vi "multiplexer timing.vi"(2 "clock time in ms (25)":u32=25, 3 "Reset":bool=TRUE) -> (1 "Clock Tick":bool, 4 "Latch":bool, 6 "Total Running Time":u32, 7 "Time Since Tick":u32, 8 "Clock Counter":u32)   [LabVIEW 2014]
panel:
  in  "latch time in ms (10)":u32
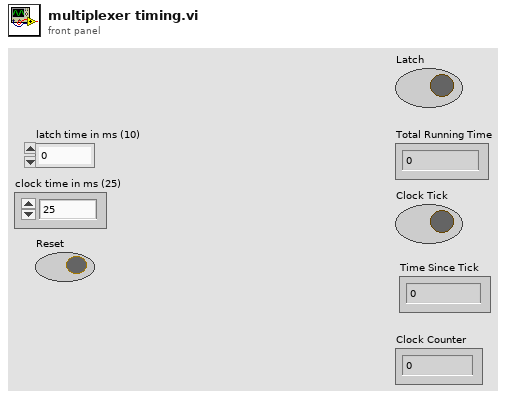
[diagram p1: front panel]
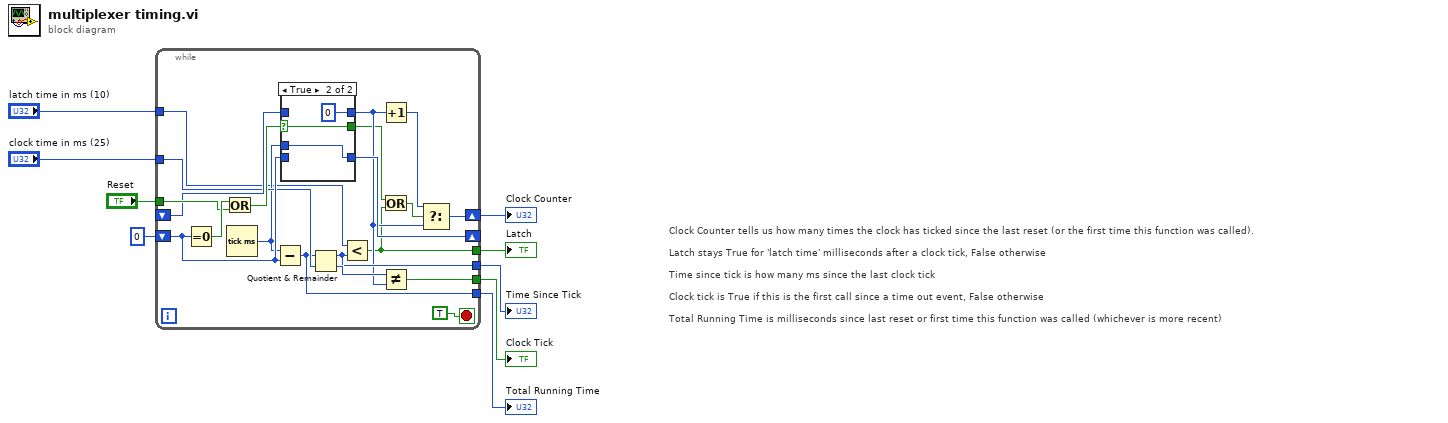
[diagram p0: block diagram]
diagram:
  # "Clock Counter tells us how many times the clock has ticked since the last reset (or the first time this function was called).\n\nLatch stays True for 'latch time' milliseconds after a clock tick, False otherwise\n\nTime since tick is how many ms since the last clock tick\n\nClock tick is True if this is the first call since a time out event, False otherwise\n\nTotal Running Time is milliseconds since last reset or first time this function was called (whichever is more recent)"
  n1 = while {
    shift-right: [w14] -> w3
    shift-left: _ -> [w22]
    shift-right: [w27] -> _
    shift-left: u32 0 -> [w26]
    tunnel: "Reset" -> [w24]
    tunnel: "clock time in ms (25)" -> [w21]
    tunnel: [w11] -> w6
    tunnel: [w18] -> w5
    tunnel: [w20] -> w4
    tunnel: "latch time in ms (10)" -> [w17]
    tunnel: [w13] -> w1
    stop <- TRUE stop-if-true
    n2 = Equal To 0?(x=w26) -> (x = 0?=w25:bool)
    n3 = Or(x=w25, y=w24) -> (x .or. y?=w23:bool)
    n4 = Tick Count (ms)() -> (millisecond timer value=w19:u32)
    n5 = Subtract(x=w19, y=w26) -> (x-y=w20:u32)
    n6 = case shown="True" w23 {
      selector: w23 -> [w30 w33]
      tunnel: [w32 w34] -> w27
      tunnel: w26 -> [w32 _]
      tunnel: w22 -> [w31 _]
      tunnel: [w31 u32 0 ("Clock Counter")] -> w15
      tunnel: w19 -> [_ w34]
      tunnel: [w30 w33] -> w12
      frame False {
      }
      frame True {
      }
    }
    n7 = Quotient & Remainder(x=w20, y=w21) -> (x-y*floor(x/y)=w18:u32, floor(x/y)=w29:u32)
    n8 = Less?(x=w17, y=w18) -> (x < y?=w13:bool)
    n9 = Increment(x=w15) -> (x+1=w16:u32)
    n10 = Or(x=w12, y=w13) -> (x .or. y?=w10:bool)
    n11 = Not Equal?(x=w29, y=w15) -> (x != y?=w11:bool)
    n12 = Select(t=w16, s=w10, f=w15) -> (s? t:f=w14:u32)
  }
  "Clock Counter" <- w3
  "Time Since Tick" <- w5
  "Clock Tick" <- w6
  "Total Running Time" <- w4
  "Latch" <- w1
